vi "ReadFile.vi"(2 "Record Folder":path=path "C:/ARC") -> (0 "CmdRes Array":string[](array[string]), 3 "Version":string, 4 "Resp. Array":string[](array[string]), 5 "Send Array":string[](array[string]), 6 "character string":string)   [LabVIEW 2017]
panel:
  out "Array":string[](array[string])
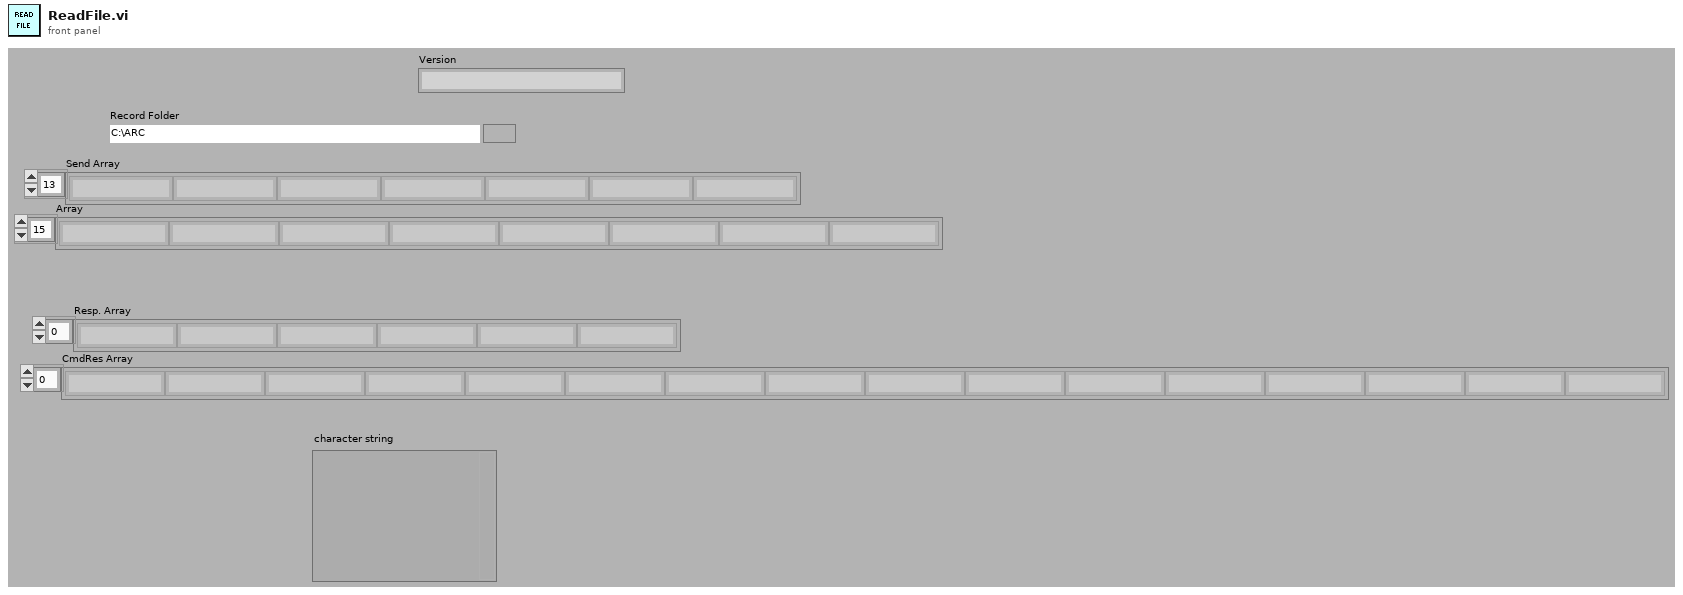
[diagram p1: front panel]
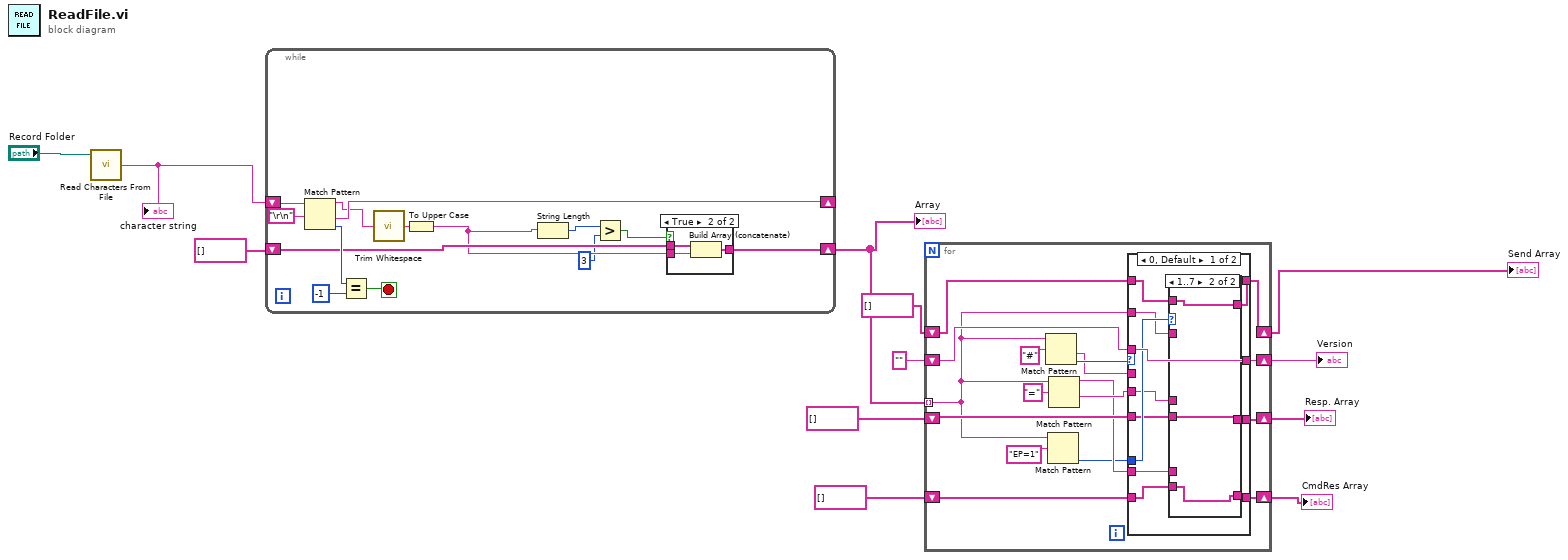
[diagram p0: block diagram]
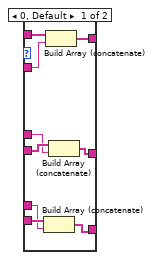
[diagram p2: hidden frame]
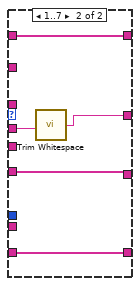
[diagram p3: hidden frame]
diagram:
  n1 = call <vilib>:"Read Characters From File.vi"("file path (dialog if empty)"="Record Folder") -> ("character string"=w11:string)  [unwired: 5 in, 3 out]
  "character string" <- w11
  n2 = while {
    shift-right: [w23] -> _
    shift-left: w11 -> [w24]
    shift-right: [w19] -> w3
    shift-left: string[] [] -> [w20]
    stop <- w25 stop-if-true
    n3 = Match Pattern(string=w24, regular expression="\r\n") -> (before substring=w21:string, after substring=w23:string, offset past match=w22:i32)  [unwired: 1 in, 1 out]
    n4 = Equal?(x=w22, y=-1) -> (x = y?=w25:bool)
    n5 = call <vilib>:"Trim Whitespace.vi"("string"=w21) -> ("trimmed string"=w18:string)  [unwired: 1 in]
    n6 = To Upper Case(1:w18) -> (0:w16:string)
    n7 = String Length(string=w16) -> (length=w15:i32)
    n8 = Greater?(x=w15, y=3) -> (0:w13:bool)
    n9 = case shown="True" w13 {
      tunnel: w20 -> [w27 w30]
      tunnel: [w27 w29] -> w19
      tunnel: w16 -> [_ w28]
      frame False {
      }
      frame True {
        n10 = Build Array (concatenate)(w30, w28) -> (w29:string[])
      }
    }
  }
  "Array" <- w3
  n11 = for {
    tunnel: w3 -> [w33] mode=indexing
    shift-right: [w40] -> w8
    shift-left: string[] [] -> [w41]
    shift-right: [w37] -> w6
    shift-left: string[] [] -> [w38]
    shift-right: [w43] -> w4
    shift-left: "" -> [w44]
    shift-right: [w31] -> w2
    shift-left: string[] [] -> [w32]
    n12 = Match Pattern(string=w33, regular expression="#") -> (after substring=w45:string, offset past match=w46:i32)  [unwired: 1 in, 2 out]
    n13 = Match Pattern(string=w33, regular expression="EP=1") -> (offset past match=w34:i32)  [unwired: 1 in, 3 out]
    n14 = Match Pattern(string=w33, regular expression="=") -> (before substring=w39:string, after substring=w42:string)  [unwired: 1 in, 2 out]
    n15 = case shown="0, Default" w46 {
      tunnel: w45 -> [_ w75]
      tunnel: w44 -> [w58 _]
      tunnel: [w58 w74] -> w43
      tunnel: w42 -> [w52 _]
      tunnel: w41 -> [w53 w73]
      tunnel: [w51 w73] -> w40
      tunnel: w39 -> [w49 _]
      tunnel: w38 -> [w50 w72]
      tunnel: [w48 w72] -> w37
      tunnel: w34 -> [w57 _]
      tunnel: w33 -> [w56 _]
      tunnel: w32 -> [w55 w71]
      tunnel: [w54 w71] -> w31
      frame 0, Default {
        n16 = case shown="1..7" w57 {
          tunnel: w56 -> [w66 _]
          tunnel: w55 -> [w67 w70]
          tunnel: [w65 w70] -> w54
          tunnel: w53 -> [w64 w69]
          tunnel: w52 -> [w63 _]
          tunnel: [w62 w69] -> w51
          tunnel: w50 -> [w61 w68]
          tunnel: w49 -> [w60 _]
          tunnel: [w59 w68] -> w48
          frame 0, Default {
            n17 = Build Array (concatenate)(w61, w60) -> (w59:string[])
            n18 = Build Array (concatenate)(w67, w66) -> (w65:string[])
            n19 = Build Array (concatenate)(w64, w63) -> (w62:string[])
          }
          frame 1..7 {
          }
        }
      }
      frame 1..7 {
        n20 = call <vilib>:"Trim Whitespace.vi"("string"=w75) -> ("trimmed string"=w74:string)  [unwired: 1 in]
      }
    }
  }
  "Send Array" <- w2
  "Resp. Array" <- w8
  "CmdRes Array" <- w6
  "Version" <- w4
